vi "Actor Core.vi"(8 "error in":errorcluster, 11 "Nested in":refnum<class "DisplayerUI.lvclass">) -> (0 "error out":errorcluster, 3 "Actor out":refnum<class "Actor.lvclass">)   [LabVIEW 2020, in "DisplayerUI.lvlib" / "DisplayerUI.lvclass"]
doc: "(<B>Filename</B>: Actor Framework.lvlib:Actor.lvclass:Actor Core.vi)\n\nReceives messages to the actor, reacts to them, and initiates any error handling that may shut the actor down.\n\nDescendant classes may override this VI to append parallel tasks for the actor to complete while it handles messages. Overrides use the Call Parent Method node."
uses:
  DisplayerUI.lvclass
  C:/Program Files/National Instruments/LabVIEW 2020/vi.lib/ActorFramework/Actor/Actor.lvclass
  <vilib>/ActorFramework/Actor/Actor.lvclass
  DisplayerUI.lvclass/DisplayerUI.ctl
  <vilib>/ActorFramework/Actor/Actor.lvclass/Actor.ctl
  <vilib>/ActorFramework/Message Enqueuer/Message Enqueuer.lvclass/Message Enqueuer.ctl
  Hardware Abstraction Layer/Component/Device/Device/DataExchange.ctl
  Interface/DataListener Messages/OnDataChange Msg/OnDataChange Msg.lvclass/OnDataChange Msg.ctl
  DisplayerUI Messages/PrepareAndSendSetROI Msg/PrepareAndSendSetROI Msg.lvclass/PrepareAndSendSetROI Msg.ctl
  <vilib>/Utility/miscctls.llb/LVRangeTypeDef.ctl
  <vilib>/ActorFramework/Message Enqueuer/Init from Existing Queue.vi
  <vilib>/ActorFramework/Message Enqueuer/Enqueue.vi
  Interface/DataListener Messages/OnDataChange Msg/OnDataChange Msg.lvclass
  C:/Program Files/National Instruments/LabVIEW 2020/vi.lib/ActorFramework/Message/Message.lvclass
  DisplayerUI Messages/PrepareAndSendSetROI Msg/PrepareAndSendSetROI Msg.lvclass
  <vilib>/ActorFramework/Stop Msg/Stop Msg.lvclass
  <vilib>/ActorFramework/Message Priority Queue/Priority Enqueue.vi
  <vilib>/ActorFramework/Message Enqueuer/Message Enqueuer.lvclass
  Hardware Abstraction Layer/Component/GenericActor/GenericActor/GenericController.lvclass
  <vilib>/vision/NI_Vision_Development_Module.lvlib
  Interface/DataListener/DataListener.lvclass
panel:
  out "RemainingTime(min)":dbl caption="Time Left((min)" format="%#.1g"
  out "AcqStatus":sgl(slide) scale=0.0..10.0 scale format="%#.1f"
  out "Max":dbl
  out "Min":dbl
  in  "Display Max":dbl
  in  "Display Min":dbl
  out "ImgIndex":dbl
  out "FPS":dbl
  in  "Threshold":cluster{i16, i16}(slide)={500, 0} scale=0.0..4096.0
  in  "Autostretch":bool
  in  "ZoomToFit":bool
  in  "Full":bool
  in  "Crop":bool
  in  "Scale Bar/um":bool
  in  "ScaleBarSize":dbl min=0.0 max=50.0
  out "RawImage":T1(plugin-control)
  # "-"
  # "-"
  # "Display Range"
  # "TH"
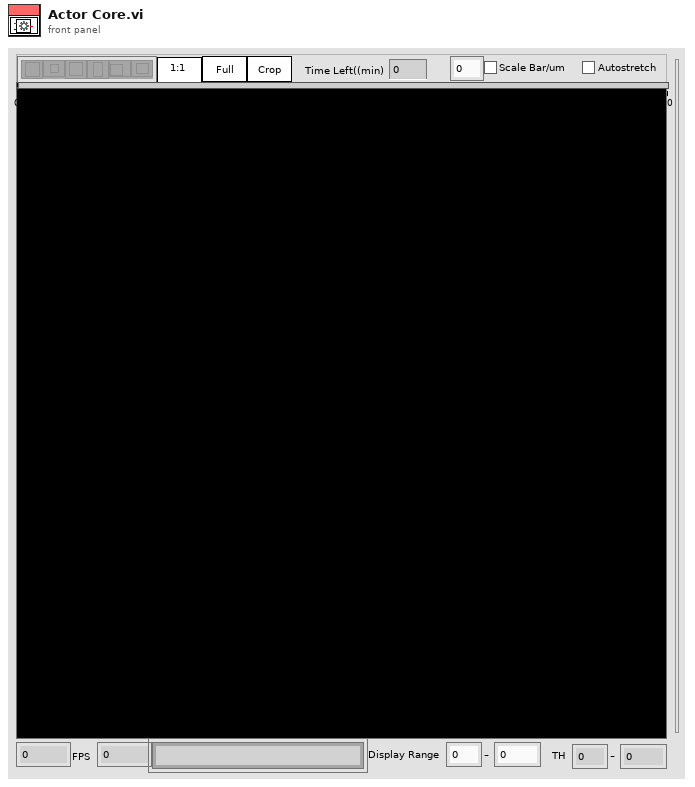
[diagram p1: front panel]
types:
  T1 = typedef "IMAQ Image.ctl" = refnum<image>
  T2 = cluster{"Stop":refnum<user-event>, "DisplayImage":refnum<user-event>}
  T3 = typedef "DataListener.lvclass/DataExchange.ctl" = cluster{"Source":string, "Destination":string, "Description":string, "value":variant}
  T4 = cluster{"Global Rectangle":i32[], "Contours":cluster{"Contour Type":u32, "ROI Type":u32, "Points":i32[]}[]}
  T5 = typedef "LVRangeTypeDef.ctl" = cluster{"Minimum":dbl, "Maximum":dbl, "Increment":dbl, "Minor Increment":dbl, "Start":dbl}
  T6 = cluster{"[0]":i32, "[1]":i32, "[2]":i32, "[3]":i32, "[4]":i32, "[5]":i32}
  T7 = cluster{"Min":sgl, "Max":sgl, "Mean":sgl, "Std Dev":sgl, "Count":i32}
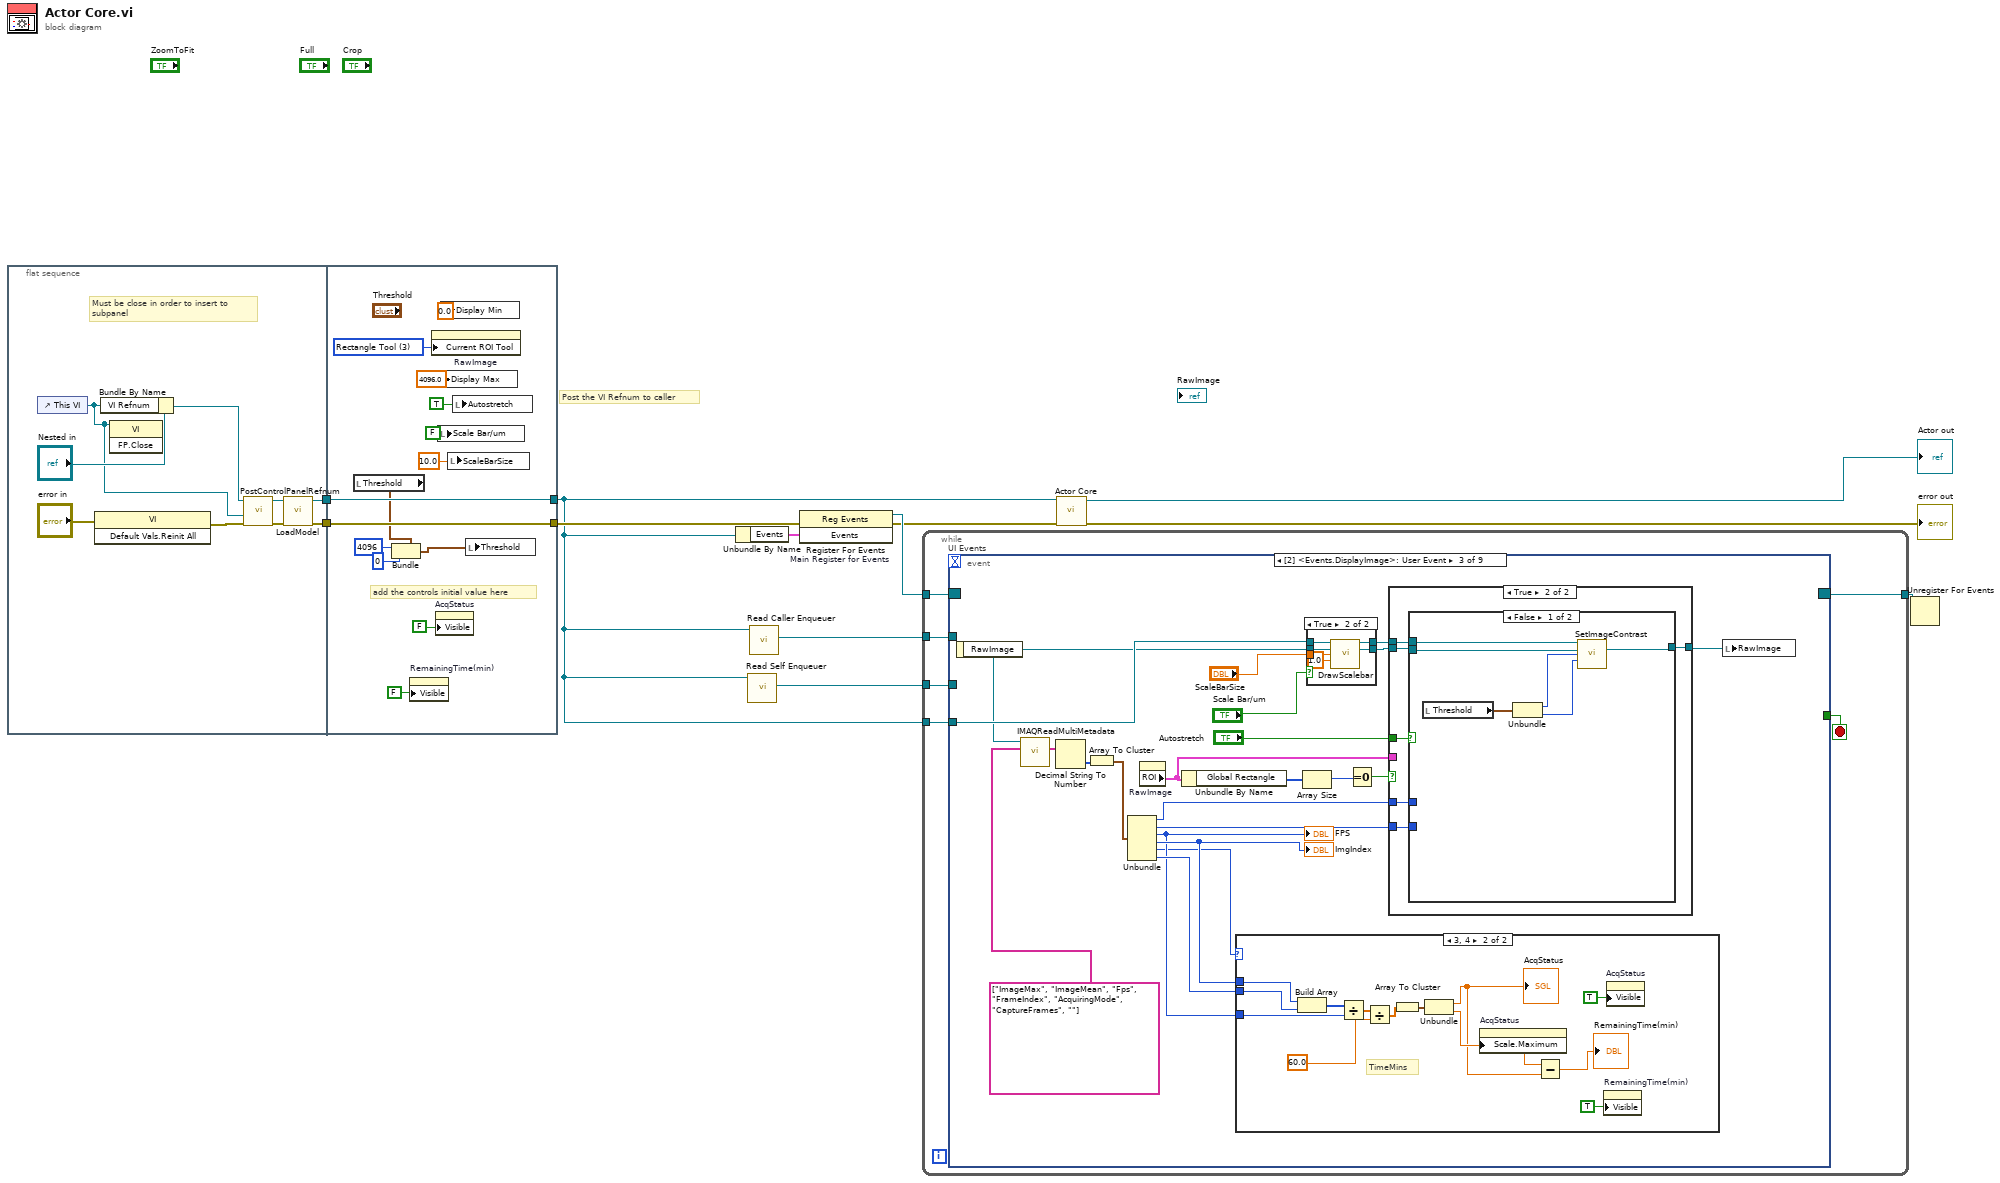
[diagram p0: block diagram]
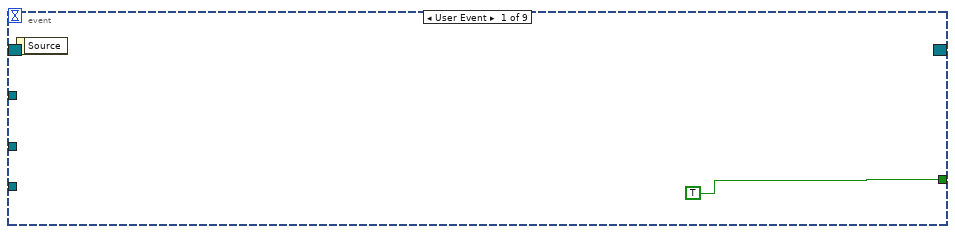
[diagram p2: hidden frame]
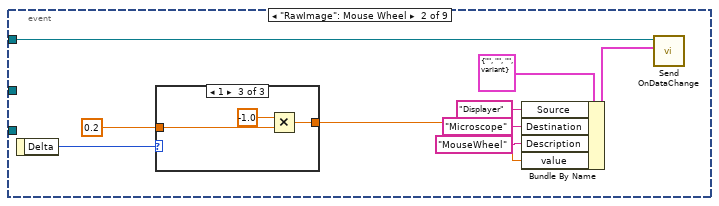
[diagram p3: hidden frame]
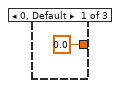
[diagram p4: hidden frame]
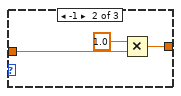
[diagram p5: hidden frame]
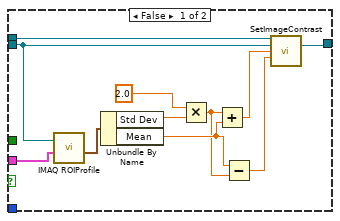
[diagram p6: hidden frame]
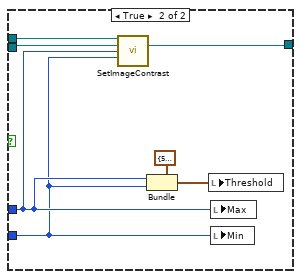
[diagram p7: hidden frame]
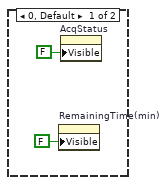
[diagram p8: hidden frame]
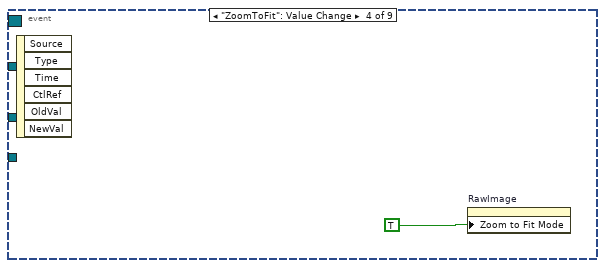
[diagram p10: hidden frame]
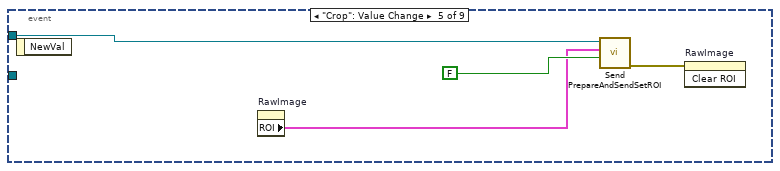
[diagram p11: hidden frame]
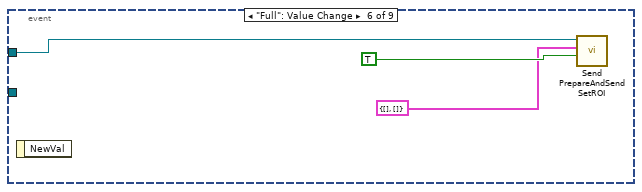
[diagram p12: hidden frame]
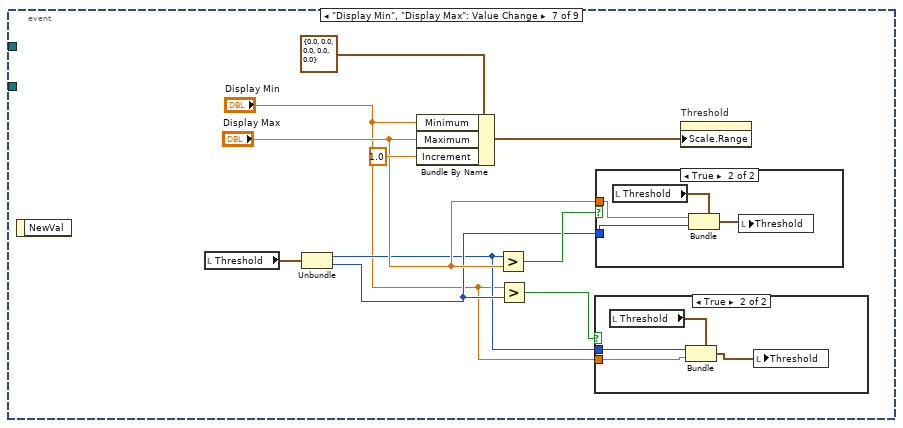
[diagram p13: hidden frame]
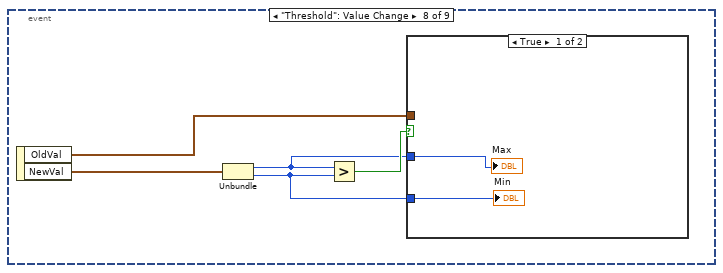
[diagram p16: hidden frame]
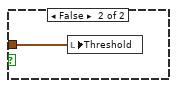
[diagram p17: hidden frame]
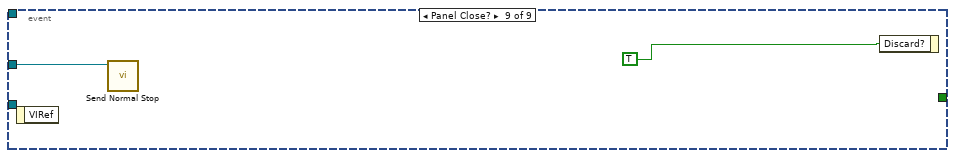
[diagram p18: hidden frame]
diagram:
  # "Post the VI Refnum to caller"
  n1 = flat-sequence {
    tunnel: [w15] -> w5
    tunnel: [w13] -> w4
    tunnel: [w34] -> w2
    tunnel: [w35] -> w3
    tunnel: w5 -> [w35]
    tunnel: w4 -> [w34]
    frame #0 {
      # "Must be close in order to insert to\nsubpanel"
      n2 = control-ref of="This VI"() -> (w16:refnum<vi>)
      n3 = invoke class="VI" method="Default Vals.Reinit All"(error in="error in") -> (error out=w19:errorcluster)  [unwired: 2 in, 2 out]
      n4 = Bundle By Name(cluster="Nested in", "VI Refnum"=w16) -> (w17:refnum<class "DisplayerUI.lvclass">)
      n5 = invoke class="VI" method="FP.Close"(reference=w16) -> ()  [unwired: 2 in, 3 out]
      n6 = call-dynamic "PostControlPanelRefnum.vi"("error in (no error)"=w19, "VI Refnum"=w16, "GRMActor in"=w17) -> ("error out"=w18:errorcluster, "GRMActor out"=w14:refnum<class "DisplayerUI.lvclass">)  [unwired: 7 in]
      n7 = call-dynamic "LoadModel.vi"("error in (no error)"=w18, "GRMActor in"=w14) -> ("error out"=w15:errorcluster, "GRMActor out"=w13:refnum<class "DisplayerUI.lvclass">)  [unwired: 8 in]
    }
    frame #1 {
      w24 = u32 3 items=["Zoom Tool"=8, "Selection Tool"=0, "Pan Tool"=9, "Point Tool"=1, "Line Tool"=2, "Rectangle Tool"=3, "Rotated Rectangle Tool"=12, "Polyline Tool"=10, "Polygon Tool"=5, "Freehand Tool"=11, "Closed Freehand Tool"=6, "Ellipse Tool"=4, "Annulus Tool"=7] ("Current ROI Tool")
      # "add the controls initial value here"
      n8 = local read "Threshold"() -> (w29:cluster{i16, i16})
      n9 = Bundle(cluster=w29, i16 4096, i16 0) -> (w30:cluster{i16, i16})
      n10 = property on="RemainingTime(min)" class="DigNum (strict)"("Visible"=FALSE) -> ()  [unwired: 2 in, 2 out]
      n11 = property on="RawImage" class="ImageControl"("Current ROI Tool"=w24) -> ()  [unwired: 2 in, 2 out]
      n12 = local write "Display Max"(4096.0 ("Max")) -> ()
      n13 = property on="AcqStatus" class="Slide (strict)"("Visible"=FALSE) -> ()  [unwired: 2 in, 2 out]
      n14 = local write "Scale Bar/um"(FALSE ("Scale Bar")) -> ()
      n15 = local write "Display Min"(0.0 ("Min")) -> ()
      n16 = local write "ScaleBarSize"(10.0 ("ScaleBarSize")) -> ()
      n17 = local write "Autostretch"(TRUE ("Autostretch")) -> ()
      n18 = local write "Threshold"(w30) -> ()
    }
  }
  n19 = Unbundle By Name(w2) -> ("Events"=w9:T2)
  n20 = call <vilib>:"Read Self Enqueuer.vi"("Actor"=w2) -> ("Self Enqueuer"=w7:refnum<class "Message Enqueuer.lvclass">)  [unwired: 10 in]
  n21 = call <vilib>:"Read Caller Enqueuer.vi"("Actor"=w2) -> ("Caller Enqueuer"=w1:refnum<class "Message Enqueuer.lvclass">)  [unwired: 10 in]
  n22 = register-events "Main Register for Events"(error in=w3, w9) -> (reference out=w10:refnum<event-registration>, error out=w6:errorcluster)  [unwired: 1 in]
  n23 = while {
    tunnel: w10 -> [w41]
    tunnel: [w39] -> w8
    tunnel: w7 -> [w38]
    tunnel: w1 -> [w37]
    tunnel: w2 -> [w36]
    stop <- w40 stop-if-true
    n24 = event "UI Events" shown="[2] <Events.DisplayImage>: User Event" {
      selector: w41 -> [_ _ _ _ _ _ _ _ _]
      dyn-events: [_ _ _ _ _ _ _ _ _] -> w39
      timeout: _ -> [_ _ _ _ _ _ _ _ _]
      tunnel: [TRUE _ _ _ _ _ _ _ _] -> w40
      tunnel: w38 -> [_ _ _ _ w135 w139 _ _ w168]
      tunnel: w37 -> [_ w43 _ _ _ _ _ _ _]
      tunnel: w36 -> [_ _ w77 _ _ _ _ _ _]
      event User Event {
        n25 = event-data() -> ()  [unwired: 1 in, 1 out]
      }
      event "RawImage": Mouse Wheel {
        n26 = event-data() -> ("Delta"=w50:i32)  [unwired: 1 in]
        n27 = case shown="1" w50 {
          tunnel: 0.2 ("Value") -> [_ w55 w58]
          tunnel: [0.0 w53 w56] -> w44
          frame 0, Default {
          }
          frame -1 {
            n28 = Multiply(x=1.0, y=w55) -> (x*y=w53:dbl)
          }
          frame 1 {
            n29 = Multiply(x=-1.0, y=w58) -> (x*y=w56:dbl)
          }
        }
        n30 = Bundle By Name(cluster=T3 {"Source"="", "Destination"="", "Description"="", "value"=variant} ("DataExchange"), "Source"="Displayer", "Destination"="Microscope", "Description"="MouseWheel", "value"=w44) -> (w48:T3)
        n31 = call "Send OnDataChange.vi"("DataExchange"=w48, "Message Enqueuer"=w43) -> ()  [unwired: 8 in, 2 out]
      }
      event User Event {
        n32 = event-data() -> ("RawImage"=w60:T1)  [unwired: 1 in]
        n33 = call "IMAQReadMultiMetadata.vi"("Keys"=string[] ["ImageMax", "ImageMean", "Fps", "FrameIndex", "AcquiringMode", "CaptureFrames", ""], "Image In"=w60) -> ("Values"=w59:string[])  [unwired: 7 in, 2 out]
        n34 = Decimal String To Number(string=w59) -> (number=w75:i32[])  [unwired: 2 in, 1 out]
        n35 = Array To Cluster(array=w75) -> (cluster=w76:T6)
        n36 = Unbundle(w76) -> ("[0]"=w74:i32, "[1]"=w73:i32, "[2]"=w70:i32, "[3]"=w71:i32, "[4]"=w69:i32, "[5]"=w72:i32)
        "ImgIndex" <- w71
        "FPS" <- w70
        n37 = property on="RawImage" class="ImageControl"() -> ("ROI"=w62:T4)  [unwired: 2 in, 2 out]
        n38 = Unbundle By Name(w62) -> ("Global Rectangle"=w68:i32[])
        n39 = case shown="3, 4" w69 {
          tunnel: w72 -> [_ w113]
          tunnel: w71 -> [_ w114]
          tunnel: w70 -> [_ w124]
          frame 0, Default {
            n40 = property on="RemainingTime(min)" class="DigNum (strict)"("Visible"=FALSE) -> ()  [unwired: 2 in, 2 out]
            n41 = property on="AcqStatus" class="Slide (strict)"("Visible"=FALSE) -> ()  [unwired: 2 in, 2 out]
          }
          frame 3, 4 {
            # "TimeMins"
            n42 = Build Array(w114, w113) -> (w122:i32[])
            n43 = Divide(x=w122, y=w124) -> (x/y=w125:dbl[])
            n44 = Divide(x=w125, y=60.0) -> (x/y=w121:dbl[])
            n45 = Array To Cluster(array=w121) -> (cluster=w120:cluster{"[0]":dbl, "[1]":dbl})
            n46 = Unbundle(w120) -> ("[0]"=w117:dbl, "[1]"=w119:dbl)
            "AcqStatus" <- w117
            n47 = property on="AcqStatus" class="Slide (strict)"("Scale.Maximum"=w119) -> ()  [unwired: 2 in, 2 out]
            n48 = Subtract(x=w119, y=w117) -> (x-y=→"RemainingTime(min)":dbl)
            n49 = property on="RemainingTime(min)" class="DigNum (strict)"("Visible"=TRUE) -> ()  [unwired: 2 in, 2 out]
            n50 = property on="AcqStatus" class="Slide (strict)"("Visible"=TRUE) -> ()  [unwired: 2 in, 2 out]
          }
        }
        n51 = Array Size(array=w68) -> (size(s)=w67:i32)
        n52 = case shown="True" "Scale Bar/um" {
          tunnel: w77 -> [w127 w133]
          tunnel: [w127 w132] -> w66
          tunnel: w60 -> [w126 w131]
          tunnel: [w126 w130] -> w65
          tunnel: "ScaleBarSize" -> [_ w129]
          frame False {
          }
          frame True {
            n53 = call-dynamic "DrawScalebar.vi"("DisplayerUI in"=w133, "Image In"=w131, "ScaleBarSize"=w129, "Binning"=1.0) -> ("DisplayerUI out"=w132:refnum<class "DisplayerUI.lvclass">, "Image Out"=w130:T1)  [unwired: 9 in, 1 out]
          }
        }
        n54 = Equal To 0?(x=w67) -> (x = 0?=w63:bool)
        n55 = case shown="True" w63 {
          tunnel: "Autostretch" -> [_ w97]
          tunnel: w74 -> [_ w96]
          tunnel: w73 -> [_ w95]
          tunnel: w66 -> [w91 w94]
          tunnel: w65 -> [w89 w93]
          tunnel: [w87 w92] -> w64
          tunnel: w62 -> [w90 _]
          frame False {
            n56 = call "IMAQ ROIProfile"("ROI Descriptor"=w90, "Image"=w89) -> ("ROI Pixel Statistics"=w88:T7)  [unwired: 2 in, 4 out]
            n57 = Unbundle By Name(w88) -> ("Std Dev"=w86:sgl, "Mean"=w83:sgl)
            n58 = Multiply(x=sgl 2.0, y=w86) -> (x*y=w82:sgl)
            n59 = Add(x=w82, y=w83) -> (x+y=w84:sgl)
            n60 = Subtract(x=w83, y=w82) -> (x-y=w81:sgl)
            n61 = call-dynamic "SetImageContrast.vi"("DisplayerUI in"=w91, "Image In"=w89, "Max"=w84, "Min"=w81) -> ("Image Dst Out"=w87:T1)  [unwired: 9 in, 2 out]
          }
          frame True {
            n62 = case shown="False" w97 {
              tunnel: w96 -> [_ w109]
              tunnel: w95 -> [_ w108]
              tunnel: w94 -> [w102 w107]
              tunnel: w93 -> [w101 w106]
              tunnel: [w98 w105] -> w92
              frame False {
                n63 = local read "Threshold"() -> (w103:cluster{i16, i16})
                n64 = Unbundle(w103) -> (w100:i16, w99:i16)
                n65 = call-dynamic "SetImageContrast.vi"("DisplayerUI in"=w102, "Image In"=w101, "Max"=w100, "Min"=w99) -> ("Image Dst Out"=w98:T1)  [unwired: 9 in, 2 out]
              }
              frame True {
                n66 = call-dynamic "SetImageContrast.vi"("DisplayerUI in"=w107, "Image In"=w106, "Max"=w109, "Min"=w108) -> ("Image Dst Out"=w105:T1)  [unwired: 9 in, 2 out]
                n67 = Bundle(cluster=cluster{i16, i16} {500, 0} ("Threshold"), w109, w108) -> (w110:cluster{i16, i16})
                n68 = local write "Threshold"(w110) -> ()
                n69 = local write "Max"(w109) -> ()
                n70 = local write "Min"(w108) -> ()
              }
            }
          }
        }
        n71 = local write "RawImage"(w64) -> ()
      }
      event "ZoomToFit": Value Change {
        n72 = event-data() -> ()  [unwired: 1 in, 6 out]
        n73 = property on="RawImage" class="ImageControl"("Zoom to Fit Mode"=TRUE) -> ()  [unwired: 2 in, 2 out]
      }
      event "Crop": Value Change {
        n74 = event-data() -> ()  [unwired: 1 in, 1 out]
        n75 = property on="RawImage" class="ImageControl"() -> ("ROI"=w137:T4)  [unwired: 2 in, 2 out]
        n76 = call "Send PrepareAndSendSetROI.vi"("Clear ROI?(F)"=FALSE, "ROI"=w137, "Message Enqueuer"=w135) -> ("error out"=w136:errorcluster)  [unwired: 7 in, 1 out]
        n77 = invoke on="RawImage" class="ImageControl" method="Clear ROI"(error in=w136) -> ()  [unwired: 2 in, 3 out]
      }
      event "Full": Value Change {
        n78 = event-data() -> ()  [unwired: 1 in, 1 out]
        n79 = call "Send PrepareAndSendSetROI.vi"("Clear ROI?(F)"=TRUE, "ROI"=T4 {"Global Rectangle"=[], "Contours"=[]}, "Message Enqueuer"=w139) -> ()  [unwired: 7 in, 2 out]
      }
      event "Display Min", "Display Max": Value Change {
        n80 = event-data() -> ()  [unwired: 1 in, 1 out]
        n81 = local read "Threshold"() -> (w148:cluster{i16, i16})
        n82 = Unbundle(w148) -> (w143:i16, w144:i16)
        n83 = Bundle By Name(cluster=T5 {"Minimum"=0.0, "Maximum"=0.0, "Increment"=0.0, "Minor Increment"=0.0, "Start"=0.0} ("Scale.Range"), "Minimum"="Display Min", "Maximum"="Display Max", "Increment"=1.0) -> (w150:T5)
        n84 = Greater?(x=w143, y="Display Max") -> (0:w147:bool)
        n85 = Greater?(x="Display Min", y=w144) -> (0:w146:bool)
        n86 = case shown="True" w146 {
          tunnel: w143 -> [_ w153]
          tunnel: "Display Min" -> [_ w152]
          frame False {
          }
          frame True {
            n87 = local read "Threshold"() -> (w155:cluster{i16, i16})
            n88 = Bundle(cluster=w155, w153, w152) -> (w154:cluster{i16, i16})
            n89 = local write "Threshold"(w154) -> ()
          }
        }
        n90 = case shown="True" w147 {
          tunnel: "Display Max" -> [_ w157]
          tunnel: w144 -> [_ w156]
          frame False {
          }
          frame True {
            n91 = local read "Threshold"() -> (w159:cluster{i16, i16})
            n92 = Bundle(cluster=w159, w157, w156) -> (w158:cluster{i16, i16})
            n93 = local write "Threshold"(w158) -> ()
          }
        }
        n94 = property on="Threshold" class="Slide (strict)"("Scale.Range"=w150) -> ()  [unwired: 2 in, 2 out]
      }
      event "Threshold": Value Change {
        n95 = event-data() -> ("OldVal"=w162:cluster{i16, i16}, "NewVal"=w164:cluster{i16, i16})  [unwired: 1 in]
        n96 = Unbundle(w164) -> (w161:i16, w160:i16)
        n97 = Greater?(x=w161, y=w160) -> (0:w163:bool)
        n98 = case shown="True" w163 {
          tunnel: w162 -> [_ w167]
          tunnel: w161 -> [w166 _]
          tunnel: w160 -> [w165 _]
          frame True {
            "Min" <- w165
            "Max" <- w166
          }
          frame False {
            n99 = local write "Threshold"(w167) -> ()
          }
        }
      }
      event Panel Close? {
        n100 = event-data() -> ()  [unwired: 1 in, 1 out]
        n101 = call <vilib>:"Send Normal Stop.vi"("Message Enqueuer"=w168) -> ()  [unwired: 10 in, 1 out]
        n102 = event-data("Discard?"=TRUE) -> ()  [unwired: 1 in, 1 out]
      }
    }
  }
  n103 = call-parent "Actor Core.vi"("error in"=w6, "GenericController in"=w2) -> ("error out"=→"error out":errorcluster, "Actor out"=→"Actor out":refnum<class "Actor.lvclass">)  [unwired: 8 in]
  n104 = Unregister For Events(event registration refnum=w8) -> ()  [unwired: 1 in, 1 out]
